vi "ChecktheNumberOfRegisters.vi"(7 "Number of Registers":i32, 8 "error in (no error)":errorcluster, 11 "Register Values":u16[](array[numeric])) -> (0 "error out":errorcluster)   [LabVIEW 2018, in "SensorPlugins.lvlib" / "SiemensDigitalEnergyMeter.lvclass"]
doc: "This VI verifys that the number of registers values matches expectation. The expectation is based on the Measurement TextRing and can be found in the Siemens Datasheet https://www.downloads.siemens.com/download-center/Download.aspx?pos=download&fct=getasset&id1=A6V10416016."
uses:
  SiemensDigitalEnergyMeter.lvclass
  <vilib>/Utility/error.llb/Error Cluster From Error Code.vi
  <vilib>/ErrorRing/Error Ring.xnode
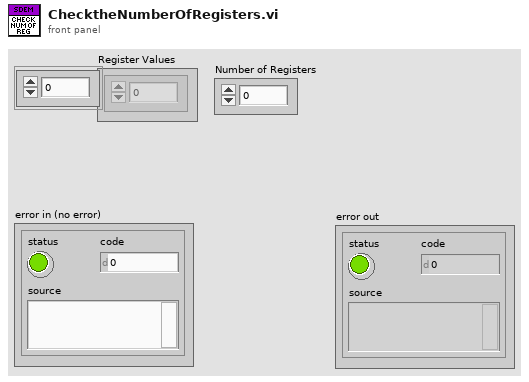
[diagram p1: front panel]
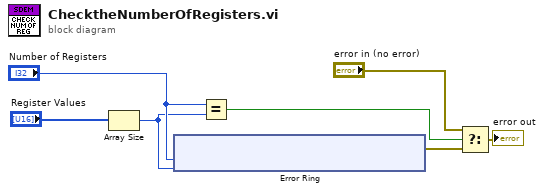
[diagram p0: block diagram]
diagram:
  n1 = Array Size(array="Register Values") -> (size(s)=w6:i32)
  n2 = xnode "Error Ring"("parameter 0"="Number of Registers", "parameter 1"=w6) -> ("error out"=w3:errorcluster)
  n3 = Equal?(x="Number of Registers", y=w6) -> (x = y?=w4:bool)
  n4 = Select(t="error in (no error)", s=w4, f=w3) -> (s? t:f=→"error out":errorcluster)
